vi "2D and 1D array for loop and while auto indexing.vi"() -> ()   [LabVIEW 2016]
panel:
  in  "stop":bool
  out "Element i":dbl
  out "B.- Random Numbers":dbl[](array[numeric])
  out "A. - Random Numbers":dbl[][](array[numeric])
  out "Column j":dbl
  out "Row i":dbl
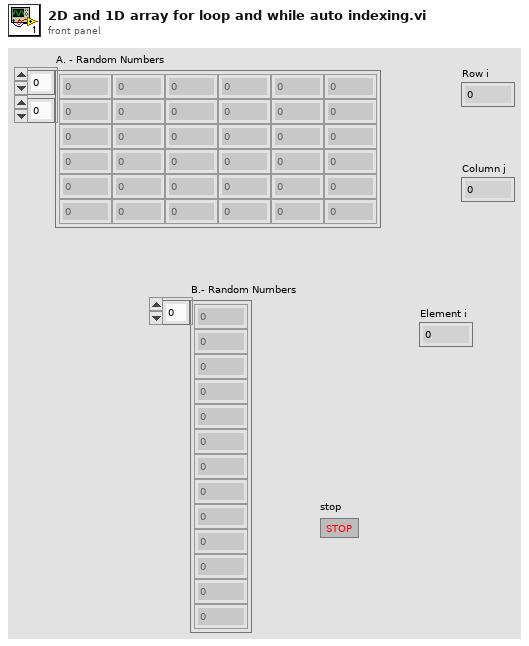
[diagram p1: front panel]
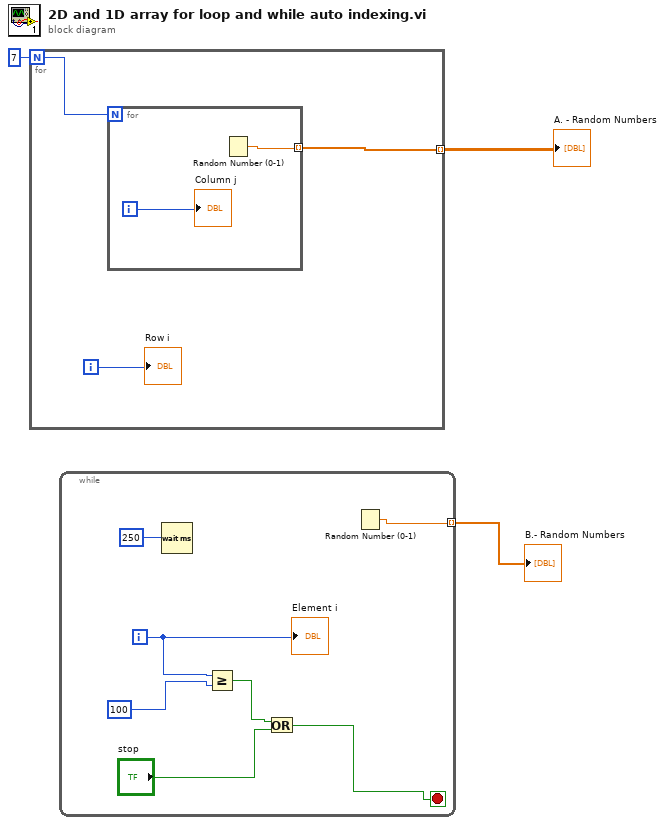
[diagram p0: block diagram]
diagram:
  n1 = for {
    N: 7 -> [w6]
    tunnel: [w4] -> w2 mode=indexing
    i -> [w5]
    n2 = for {
      N: w6 -> [_]
      tunnel: [w7] -> w4 mode=indexing
      i -> [w8]
      n3 = Random Number (0-1)() -> (number: 0 to 1=w7:dbl)
      "Column j" <- w8
    }
    "Row i" <- w5
  }
  "A. - Random Numbers" <- w2
  n4 = while {
    tunnel: [w14] -> w1 mode=indexing
    i -> [w13]
    stop <- w10 stop-if-true
    n5 = Wait (ms)(milliseconds to wait=u32 250 ("millisecond timer value")) -> ()  [unwired: 1 out]
    n6 = Greater Or Equal?(x=w13, y=u32 100 ("millisecond timer value")) -> (x >= y?=w11:bool)
    n7 = Or(x=w11, y="stop") -> (x .or. y?=w10:bool)
    n8 = Random Number (0-1)() -> (number: 0 to 1=w14:dbl)
    "Element i" <- w13
  }
  "B.- Random Numbers" <- w1
